vi "single image acquire ll.vi"(8 "Image name":string, 10 "Camera Name":refnum<k21>="cam0" caption="IMAQdx Session", 11 "File Path":path) -> (0 "Image Out":T1, 3 "Image":T1(plugin-control))   [LabVIEW 2017]
uses:
  <vilib>/vision/Image Controls.llb/IMAQ Image.ctl
  <vilib>/vision/driver/NI_Vision_Acquisition_Software.lvlib
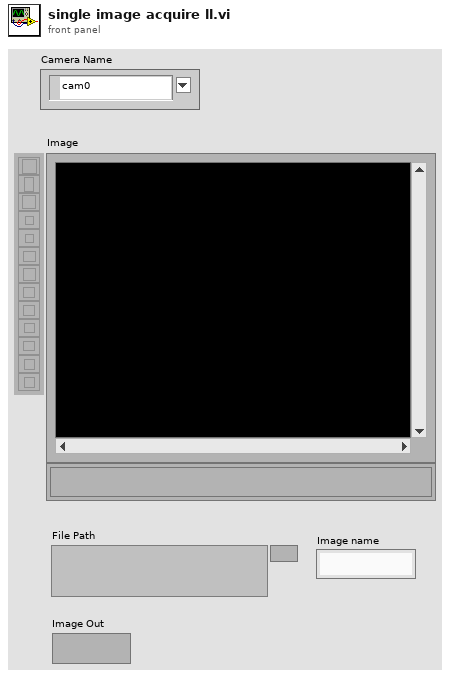
[diagram p1: front panel]
types:
  T1 = typedef "IMAQ Image.ctl" = refnum<image>
  T2 = typedef "IMAQdx.ctl" = refnum<k21>
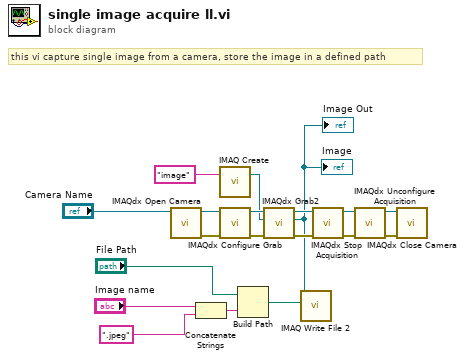
[diagram p0: block diagram]
diagram:
  # "this vi capture single image from a camera, store the image in a defined path"
  n1 = call <vilib>:"IMAQdx Open Camera.vi"("Session In"="Camera Name") -> ("error out"=w13:errorcluster, "Session Out"=w15:T2)  [unwired: 2 in, 7 out]
  n2 = Concatenate Strings("Image name", ".jpeg" ("string")) -> (w4:string)
  n3 = call "IMAQ Create"("Image Name"="image") -> ("New Image"=w10:T1)  [unwired: 3 in, 2 out]
  n4 = call <vilib>:"IMAQdx Configure Grab.vi"("error in"=w13, "Session In"=w15) -> ("error out"=w11:errorcluster, "Session Out"=w12:T2)  [unwired: 8 in]
  n5 = Build Path(base path="File Path", name or relative path=w4) -> (appended path=w3:path)
  n6 = call <vilib>:"IMAQdx Grab2.vi"("error in"=w11, "Image In"=w10, "Session In"=w12) -> ("error out"=w7:errorcluster, "Image Out"=w6:T1, "Session Out"=w8:T2)  [unwired: 5 in, 1 out]
  "Image Out" <- w6
  "Image" <- w6
  n7 = call-poly "IMAQ Write File 2"("File Path"=w3, "Image"=w6) -> ()  [unwired: 8 in, 2 out]
  n8 = call <vilib>:"IMAQdx Stop Acquisition.vi"("error in"=w7, "Session In"=w8) -> ("error out"=w16:errorcluster, "Session Out"=w17:T2)  [unwired: 8 out]
  n9 = call <vilib>:"IMAQdx Unconfigure Acquisition.vi"("error in"=w16, "Session In"=w17) -> ("error out"=w18:errorcluster, "Session Out"=w19:T2)  [unwired: 8 out]
  n10 = call <vilib>:"IMAQdx Close Camera.vi"("error in"=w18, "Session In"=w19) -> ()  [unwired: 10 out]
